vi "createBroadcastSetForceFrame.vi"(8 "error in (no error)":errorcluster, 9 "SlewFlag":bool, 10 "BroadcastCounter":u8, 11 "FAILC in":refnum<class "FAILC.lvclass">) -> (0 "error out":errorcluster, 2 "FixedFrameBuilder":refnum<class "FixedFrameBuilder.lvclass">, 3 "FAILC out":refnum<class "FAILC.lvclass">)   [LabVIEW 2016, in "RTFAILC.lvlib" / "FAILC.lvclass"]
uses:
  FAILC.lvclass
  Common_RT_Modbus/FixedFrameBuilder/FixedFrameBuilder.lvclass
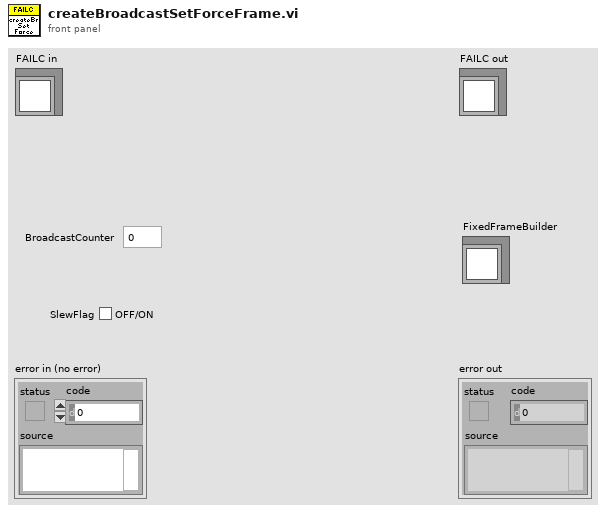
[diagram p1: front panel]
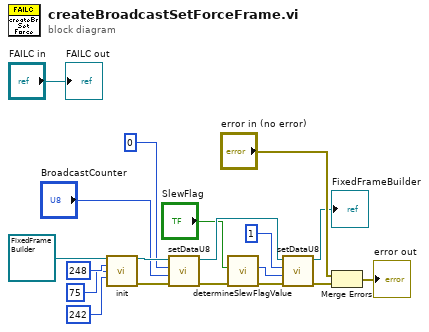
[diagram p0: block diagram]
diagram:
  n1 = call "init.vi"("FixedFrameBuilder in"=refnum<class "FixedFrameBuilder.lvclass"> refnum ("RTModbus.lvlib:FixedFrameBuilder.lvclass"), "Address"=u8 248, "Function"=u8 75, "DataSize"=242) -> ("FixedFrameBuilder out"=w15:refnum<class "FixedFrameBuilder.lvclass">, "error out"=w19:errorcluster)  [unwired: 10 in]
  n2 = call "setDataU8.vi"("error in (no error)"=w19, "Data"="BroadcastCounter", "Index"=0, "FixedFrameBuilder in"=w15) -> ("error out"=w3:errorcluster, "FixedFrameBuilder out"=w8:refnum<class "FixedFrameBuilder.lvclass">)  [unwired: 6 in]
  n3 = call "determineSlewFlagValue.vi"("error in (no error)"=w3, "SlewFlag"="SlewFlag") -> ("error out"=w2:errorcluster, "FlagValue"=w1:u8)  [unwired: 7 in, 1 out]
  n4 = call "setDataU8.vi"("error in (no error)"=w2, "Data"=w1, "Index"=1, "FixedFrameBuilder in"=w8) -> ("error out"=w6:errorcluster, "FixedFrameBuilder out"=→"FixedFrameBuilder":refnum<class "FixedFrameBuilder.lvclass">)  [unwired: 6 in]
  n5 = Merge Errors("error in (no error)", w6) -> (→"error out":errorcluster)
  "FAILC out" <- "FAILC in"
